vi "comm wait for event.vi"(8 "error in (no error)":errorcluster, 10 "milliseconds timeout":u32, 11 "Comm Handle":u64) -> (0 "error out":errorcluster, 2 "event mask":u32, 3 "dup Comm Handle":u64)   [LabVIEW 2009, in "lvserial.lvlib"]
doc: "Waits for an event to occur for a specified communications device."
uses:
  lvserial.lvlib
  x64/Release/lvserial.dll
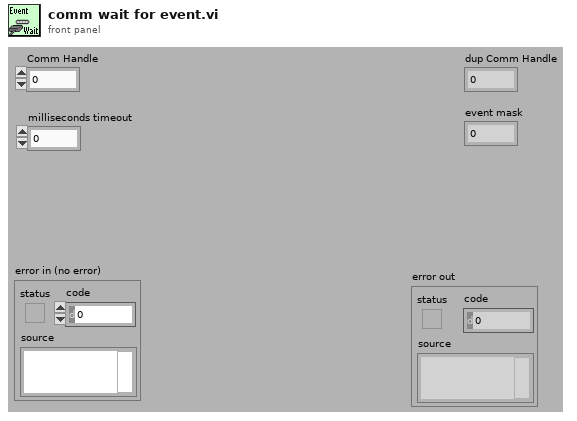
[diagram p1: front panel]
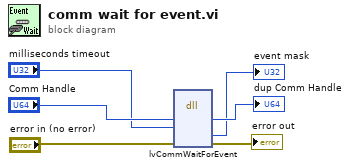
[diagram p0: block diagram]
diagram:
  n1 = dll-call lib="C:/Users/Admin/Desktop/lvserial_source_1-2-13/x64/Release/lvserial.dll" fn="lvCommWaitForEvent"("hComm"="Comm Handle", "ulTimeout"="milliseconds timeout", "error"="error in (no error)") -> ("hComm"=→"dup Comm Handle":u64, "pulEventMask"=→"event mask":u32, "error"=→"error out":errorcluster)  [unwired: 5 in, 3 out]
